vi "mob_calc_subvi.vi"(5 "Width":dbl, 7 "Length":dbl, 9 "Dielectric (d)":dbl, 10 "Sat Id Used":dbl[](array[numeric]), 11 "Vg Used":dbl[](array[numeric])) -> (1 "Capacitance":dbl, 2 "Vt":dbl, 3 "Mobility":dbl)   [LabVIEW 2011]
uses:
  <vilib>/Analysis/NI_AALPro.lvlib
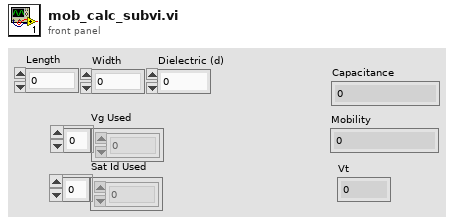
[diagram p1: front panel]
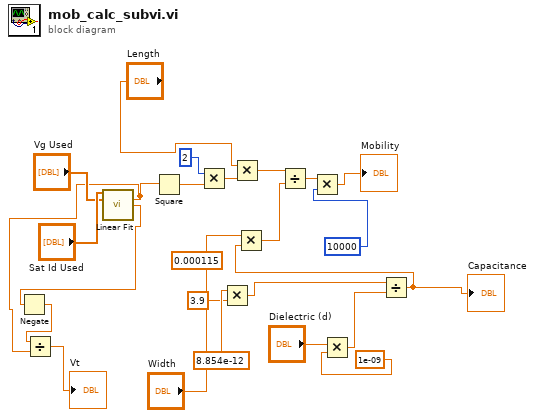
[diagram p0: block diagram]
diagram:
  (unwired) 0.000115
  n1 = call <vilib>:"Linear Fit.vi"("Y"="Sat Id Used", "X"="Vg Used") -> ("slope"=w2:dbl, "intercept"=w3:dbl)  [unwired: 9 in, 3 out]
  n2 = Negate(x=w3) -> (-x=w4:dbl)
  n3 = Divide(x=w4, y=w2) -> (x/y=→"Vt":dbl)
  n4 = Square(x=w2) -> (x^2=w15:dbl)
  n5 = Multiply(x=2, y=w15) -> (x*y=w14:dbl)
  n6 = Multiply(x=8.854e-12, y=3.9) -> (x*y=w23:dbl)
  n7 = Multiply(x="Length", y=w14) -> (x*y=w13:dbl)
  n8 = Multiply(x="Dielectric (d)", y=1e-09) -> (x*y=w22:dbl)
  n9 = Divide(x=w23, y=w22) -> (x/y=w1:dbl)
  "Capacitance" <- w1
  n10 = Multiply(x="Width", y=w1) -> (x*y=w12:dbl)
  n11 = Divide(x=w13, y=w12) -> (x/y=w10:dbl)
  n12 = Multiply(x=w10, y=10000) -> (x*y=→"Mobility":dbl)
